vi "WLAN - TV - RW - UTIL - Rx_TestVectors.vi"(0 "Rx Measurements Settings":T1[](array[typedef]) {"DSSS Data Rate (Mbps)" items=["1", "2", "5.5 CCK", "5.5 PBCC", "11 CCK", "11 PBCC", "22", "33"]; "OFDM Data Rate (Mbps)" items=["6", "9", "12", "18", "24", "36", "48", "54"]; "80211n PLCP Frame Format" items=["Mixed Format", "Greenfield Format"]; "Standard" items=["80211A/G/J/P OFDM", "80211B/G DSSS", "80211G DSSSOFDM", "80211N MIMOOFDM", "80211AC MIMOOFDM"]}) -> ()   [LabVIEW 2011]
uses:
  <vilib>/Utility/file.llb/Write To Spreadsheet File (DBL).vi
  <vilib>/Utility/file.llb/Write To Spreadsheet File (string).vi
  Includes/WLAN - TV - RW - INC - TV_Cluster.ctl
  Includes/WLAN - TV - RW - INC - TV_Rx_Measurements.ctl
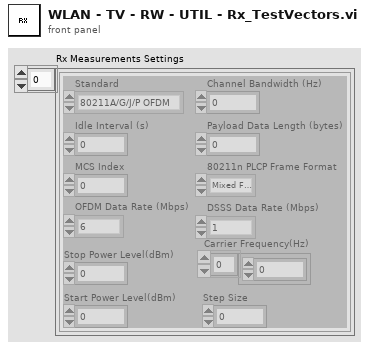
[diagram p1: front panel]
types:
  T1 = typedef "WLAN - TV - RW - INC - TV_Rx_Measurements.ctl" = cluster{"Standard":i32, "Channel Bandwidth (Hz)":dbl, "Idle Interval (s)":dbl, "MCS Index":i32, "80211n PLCP Frame Format":i32, "Payload Data Length (bytes)":i32, "OFDM Data Rate (Mbps)":i32, "DSSS Data Rate (Mbps)":i32, "Carrier Frequency(Hz)":dbl[], "Start Power Level(dBm)":dbl, "Stop Power Level(dBm)":dbl, "Step Size":dbl}
  T2 = typedef "WLAN - TV - RW - INC - TV_Cluster.ctl" = cluster{"Standard ":string, "Channel Number":string, "Channel Frequency(Hz)":string, "Power Level(milli-dBm)":string, "Power Level(dBm)":string, "Channel Bandwidth (Hz)":string, "Idle Interval (s)":string, "OFDM Data Rate (Mbps)":string, "OFDM Payload Length (bytes)":string, "Number of Packets":string, "MCS Index":string, "Guard Interval (s)":string, "80211n PLCP Frame Format":string, "FEC Coding Type":string, "DSSS Data Rate (Mbps)":string, "DSSS Payload Length (bytes)":string, "Averages":string}
  T3 = enum16{"2G Band 20M", "5G Band 20M", "5G Band 40M"}
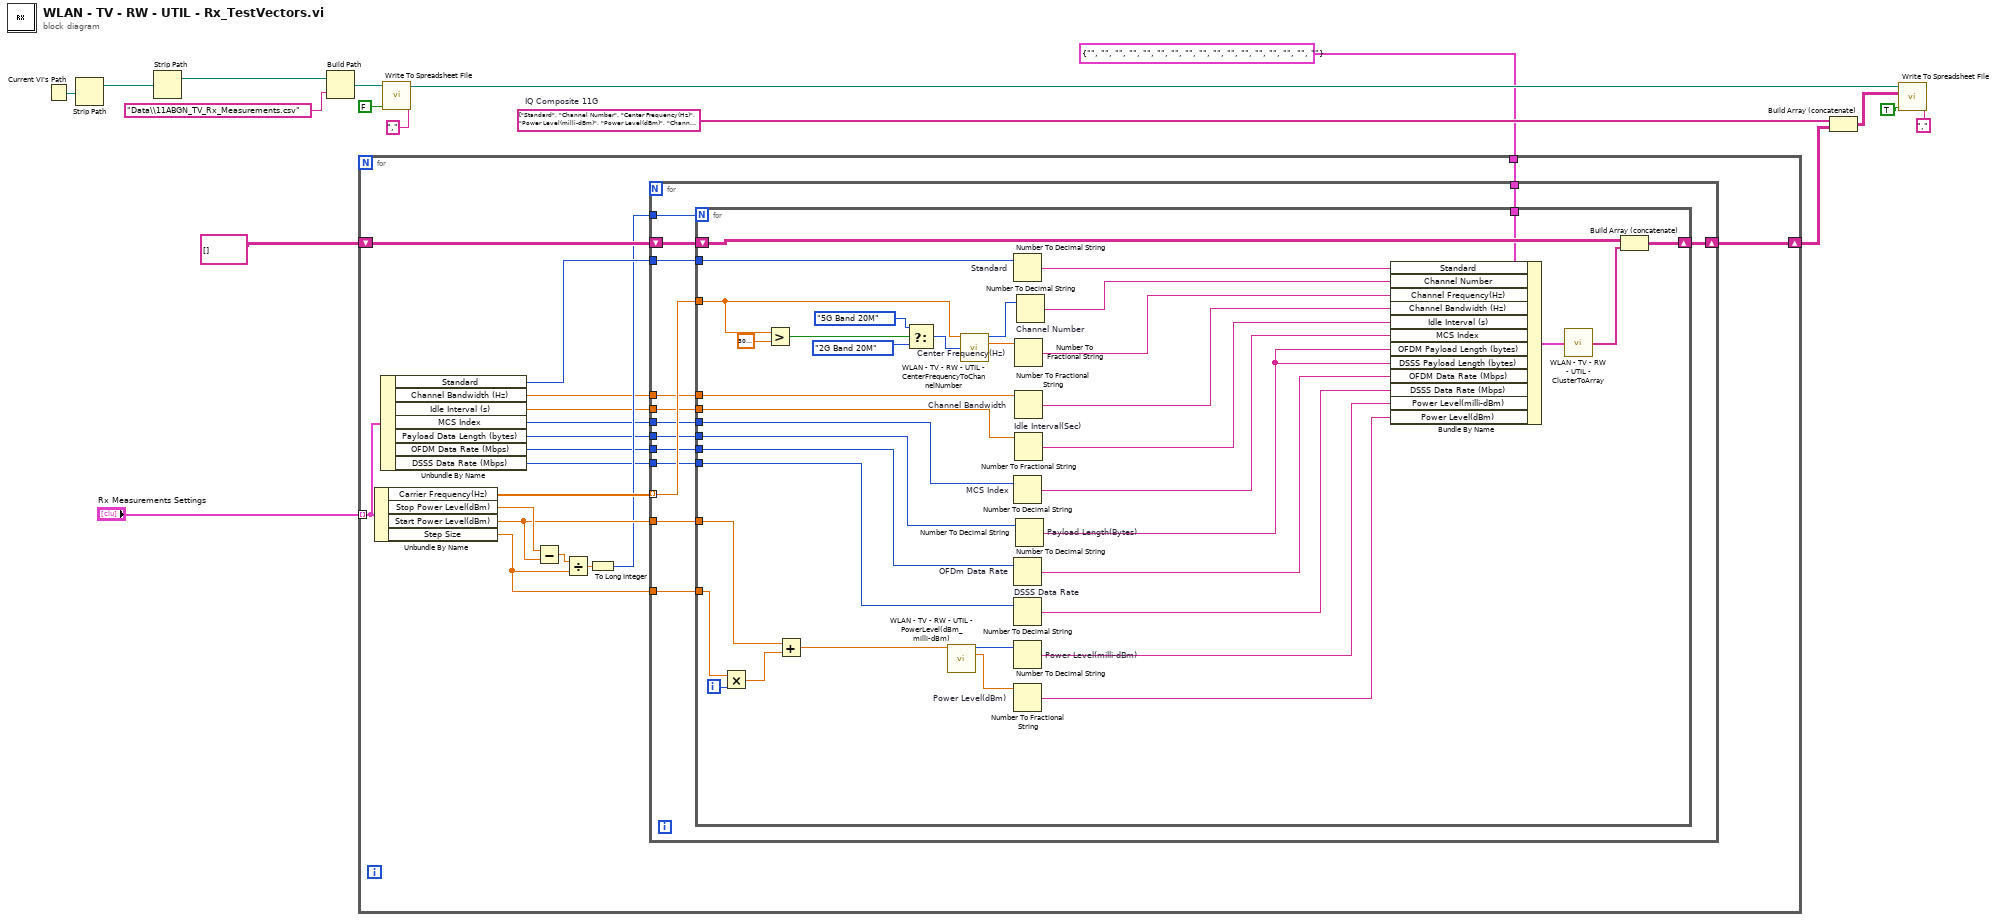
[diagram p0: block diagram]
diagram:
  w7 = string[] ["Standard", "Channel Number", "Center Frequency(Hz)", "Power Level(milli-dBm)", "Power Level(dBm)", "Channel BW(Hz)", "Idle Interval(Sec)", "OFDM Data Rate(Enum)", "OFDM Payload Length(Bytes)", "Number of Packets"]  # IQ Composite 11G
  n1 = Current VI's Path() -> (path=w16:path)
  n2 = Strip Path(path=w16) -> (stripped path=w4:path)  [unwired: 1 out]
  n3 = Strip Path(path=w4) -> (stripped path=w3:path)  [unwired: 1 out]
  n4 = Build Path(base path=w3, name or relative path="Data\\11ABGN_TV_Rx_Measurements.csv") -> (appended path=w12:path)
  n5 = for {
    shift-right: [w17] -> w6
    shift-left: string[][] [] ("appended array") -> [w34]
    tunnel: T2 {"Standard "="", "Channel Number"="", "Channel Frequency(Hz)"="", "Power Level(milli-dBm)"="", "Power Level(dBm)"="", "Channel Bandwidth (Hz)"="", "Idle Interval (s)"="", "OFDM Data Rate (Mbps)"="", "OFDM Payload Length (bytes)"="", "Number of Packets"="", "MCS Index"="", "Guard Interval (s)"="", "80211n PLCP Frame Format"="", "FEC Coding Type"="", "DSSS Data Rate (Mbps)"="", "DSSS Payload Length (bytes)"="", "Averages"=""} ("TV Paramaters") -> [w33]
    tunnel: "Rx Measurements Settings" -> [w28] mode=indexing
    n6 = Unbundle By Name(w28) -> ("Carrier Frequency(Hz)"=w32:dbl[], "Stop Power Level(dBm)"=w31:dbl, "Start Power Level(dBm)"=w26:dbl, "Step Size"=w24:dbl)
    n7 = Unbundle By Name(w28) -> ("Standard"=w27:i32, "Channel Bandwidth (Hz)"=w23:dbl, "Idle Interval (s)"=w22:dbl, "MCS Index"=w21:i32, "Payload Data Length (bytes)"=w20:i32, "OFDM Data Rate (Mbps)"=w19:i32, "DSSS Data Rate (Mbps)"=w18:i32)
    n8 = Subtract(x=w31, y=w26) -> (x-y=w30:dbl)
    n9 = Divide(x=w30, y=w24) -> (x/y=w29:dbl)
    n10 = To Long Integer(number=w29) -> (32bit integer=w25:i32)
    n11 = for {
      tunnel: w27 -> [w47]
      tunnel: w33 -> [w46]
      tunnel: w32 -> [w44] mode=indexing
      tunnel: w25 -> [w45]
      tunnel: w26 -> [w42]
      tunnel: w24 -> [w43]
      tunnel: w23 -> [w41]
      tunnel: w22 -> [w40]
      tunnel: w21 -> [w39]
      tunnel: w20 -> [w38]
      tunnel: w19 -> [w37]
      tunnel: w18 -> [w36]
      shift-right: [w35] -> w17
      shift-left: w34 -> [w48]
      n12 = for {
        N: w45 -> [_]
        tunnel: w44 -> [w67]
        shift-right: [w86] -> w35
        shift-left: w48 -> [w85]
        tunnel: w47 -> [w84]
        tunnel: w46 -> [w78]
        tunnel: w43 -> [w63]
        tunnel: w42 -> [w61]
        tunnel: w41 -> [w59]
        tunnel: w40 -> [w58]
        tunnel: w39 -> [w54]
        tunnel: w38 -> [w55]
        tunnel: w37 -> [w52]
        tunnel: w36 -> [w51]
        i -> [w64]
        n13 = Multiply(x=w63, y=w64) -> (x*y=w62:dbl)
        n14 = Greater?(x=w67, y=3000000000.0) -> (0:w65:bool)
        n15 = Add(x=w61, y=w62) -> (x+y=w60:dbl)
        n16 = Select(t=T3."5G Band 20M" ("Frequency Band"), s=w65, f=T3."2G Band 20M" ("Frequency Band")) -> (s? t:f=w69:T3)
        n17 = call "WLAN - TV - RW - UTIL - PowerLevel(dBm_milli-dBm).vi"("Power Level(dBm)"=w60) -> ("Coherced Power(milli-dBm)"=w81:i32, "Coherced Power(dBm)"=w80:dbl)  [unwired: 13 in]
        n18 = call "WLAN - TV - RW - UTIL - CenterFrequencyToChannelNumber.vi"("Center Frequency(Hz)"=w67, 7:w69) -> ("Coherced Channel Number"=w82:i32, "Coherced Center Frequency (Hz)"=w83:dbl)  [unwired: 12 in]
        n19 = Number To Decimal String "Standard"(number=w84) -> (decimal integer string=w71:string)  [unwired: 1 in]
        n20 = Number To Decimal String "MCS Index"(number=w54) -> (decimal integer string=w76:string)  [unwired: 1 in]
        n21 = Number To Decimal String "OFDm Data Rate"(number=w52) -> (decimal integer string=w50:string)  [unwired: 1 in]
        n22 = Number To Decimal String "DSSS Data Rate"(number=w51) -> (decimal integer string=w49:string)  [unwired: 1 in]
        n23 = Number To Decimal String "Power Level(milli-dBm)"(number=w81) -> (decimal integer string=w57:string)  [unwired: 1 in]
        n24 = Number To Fractional String "Power Level(dBm)"(number=w80) -> (F-format string=w56:string)  [unwired: 3 in]
        n25 = Number To Fractional String "Center Frequency(Hz)"(number=w83) -> (F-format string=w73:string)  [unwired: 3 in]
        n26 = Number To Fractional String "Channel Bandwidth"(number=w59) -> (F-format string=w74:string)  [unwired: 3 in]
        n27 = Number To Fractional String "Idle Interval(Sec)"(number=w58) -> (F-format string=w75:string)  [unwired: 3 in]
        n28 = Number To Decimal String "Payload Length(Bytes)"(number=w55) -> (decimal integer string=w53:string)  [unwired: 1 in]
        n29 = Number To Decimal String "Channel Number"(number=w82) -> (decimal integer string=w72:string)  [unwired: 1 in]
        n30 = Bundle By Name(cluster=w78, "Standard"=w71, "Channel Number"=w72, "Channel Frequency(Hz)"=w73, "Channel Bandwidth (Hz)"=w74, "Idle Interval (s)"=w75, "MCS Index"=w76, "OFDM Payload Length (bytes)"=w53, "DSSS Payload Length (bytes)"=w53, "OFDM Data Rate (Mbps)"=w50, "DSSS Data Rate (Mbps)"=w49, "Power Level(milli-dBm)"=w57, "Power Level(dBm)"=w56) -> (w77:T2)
        n31 = call "WLAN - TV - RW - UTIL - ClusterToArray.vi"("TV Paramaters"=w77) -> ("TV_Parameters(1-D array)"=w79:string[])  [unwired: 14 in]
        n32 = Build Array (concatenate)(w85, w79) -> (w86:string[][])
      }
    }
  }
  n33 = call-poly <vilib>:"Write To Spreadsheet File.vi"("delimiter (\\t)"="," ("delimiter (\\t)"), "append to file? (new file:F)"=FALSE, "file path (dialog if empty)"=w12) -> ("new file path (Not A Path if cancelled)"=w11:path)  [unwired: 5 in]
  n34 = Build Array (concatenate)(w7, w6) -> (w5:string[][])
  n35 = call-poly <vilib>:"Write To Spreadsheet File.vi"("delimiter (\\t)"="," ("delimiter (\\t)"), "append to file? (new file:F)"=TRUE, "2D data"=w5, "file path (dialog if empty)"=w11) -> ()  [unwired: 4 in, 1 out]
